vi "SetStreamingFilter.Do.vi"(8 "error in (no error)":errorcluster, 10 "State Variables":T1, 11 "gRPC Request":T12) -> (0 "error out":errorcluster, 2 "State Variables out":T1, 3 "gRPC Response":T13)   [LabVIEW 2025, in "xnet_can_bus_monitor_api_server_do.lvlib"]
uses:
  xnet_can_bus_monitor_api_server_do.lvlib
  xnet_can_bus_monitor_api_server/RPC Messages/ni_xnet_can_bm_api_ErrorInfo.ctl
  xnet_can_bus_monitor_api_server/xnet_can_bus_monitor_api_server.lvlib
  xnet_can_bus_monitor_api_server/RPC Messages/ni_xnet_can_bm_api_SetStreamingFilterReply.ctl
  xnet_can_bus_monitor_api_server/RPC Messages/ni_xnet_can_bm_api_FrameFilter.ctl
  xnet_can_bus_monitor_api_server/RPC Messages/ni_xnet_can_bm_api_DirectionFilter.ctl
  xnet_can_bus_monitor_api_server/RPC Messages/ni_xnet_can_bm_api_FilterInfo.ctl
  xnet_can_bus_monitor_api_server/RPC Messages/ni_xnet_can_bm_api_FdIsoMode.ctl
  xnet_can_bus_monitor_api_server/RPC Messages/ni_xnet_can_bm_api_Termination.ctl
  xnet_can_bus_monitor_api_server/RPC Messages/ni_xnet_can_bm_api_CanMode.ctl
  xnet_can_bus_monitor_api_server/RPC Messages/ni_xnet_can_bm_api_ConnectSettings.ctl
  Types/XNET.InitialSettings.ctl
  Types/StreamProcess.VIRef.ctl
  Types/StreamProcess.Refs.ctl
  Types/MainProcess.StateVariables.ctl
  xnet_can_bus_monitor_api_server/RPC Messages/ni_xnet_can_bm_api_SetStreamingFilterRequest.ctl
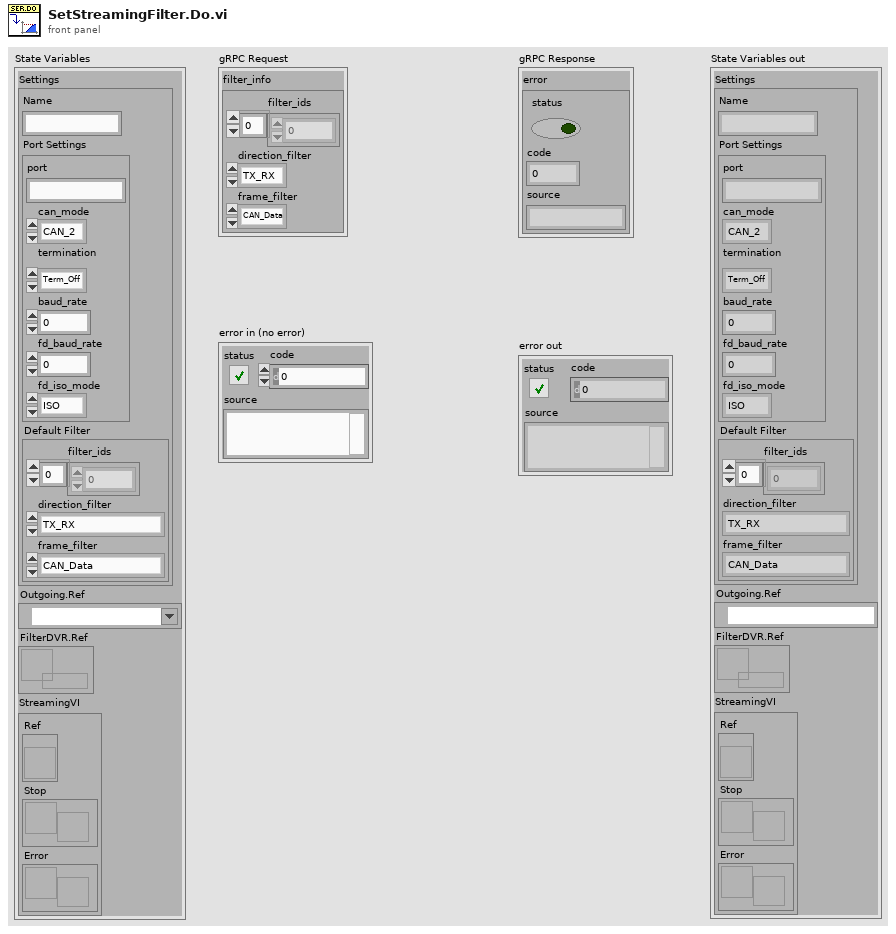
[diagram p1: front panel]
types:
  T1 = typedef "xnet_can_bus_monitor_api_server_do.lvlib/MainProcess.StateVariables.ctl" = cluster{"Settings":T2, "Outgoing.Ref":refnum<k21>, "FilterDVR.Ref":refnum<data-value>, "StreamingVI":T10}
  T2 = typedef "xnet_can_bus_monitor_api_server_do.lvlib/XNET.InitialSettings.ctl" = cluster{"Name":string, "Port Settings":T3, "Default Filter":T7}
  T3 = typedef "xnet_can_bus_monitor_api_server.lvlib/ni_xnet_can_bm_api_ConnectSettings.ctl" = cluster{"port":string, "can_mode":T4, "termination":T5, "baud_rate":u64, "fd_baud_rate":u64, "fd_iso_mode":T6}
  T4 = typedef "xnet_can_bus_monitor_api_server.lvlib/ni_xnet_can_bm_api_CanMode.ctl" = enum32{"CAN_2", "CAN_FD", "CAN_FD_BRS"}
  T5 = typedef "xnet_can_bus_monitor_api_server.lvlib/ni_xnet_can_bm_api_Termination.ctl" = enum32{"Term_Off", "Term_On"}
  T6 = typedef "xnet_can_bus_monitor_api_server.lvlib/ni_xnet_can_bm_api_FdIsoMode.ctl" = enum32{"ISO", "Non_ISO", "ISO_Legacy"}
  T7 = typedef "xnet_can_bus_monitor_api_server.lvlib/ni_xnet_can_bm_api_FilterInfo.ctl" = cluster{"filter_ids":u32[], "direction_filter":T8, "frame_filter":T9}
  T8 = typedef "xnet_can_bus_monitor_api_server.lvlib/ni_xnet_can_bm_api_DirectionFilter.ctl" = enum32{"TX_RX", "RX", "TX"}
  T9 = typedef "xnet_can_bus_monitor_api_server.lvlib/ni_xnet_can_bm_api_FrameFilter.ctl" = enum32{"CAN_Data", "CAN_Remote", "CAN_Bus_Error", "CAN_2_Data", "CAN_FD_Data", "CAN_FD_BRS_Data", "J1939_Data", "Delay", "Log_Trigger", "Start_Trigger", "All"}
  T10 = typedef "xnet_can_bus_monitor_api_server_do.lvlib/StreamProcess.Refs.ctl" = cluster{"Ref":T11, "Stop":refnum<notifier>, "Error":refnum<notifier>}
  T11 = typedef "xnet_can_bus_monitor_api_server_do.lvlib/StreamProcess.VIRef.ctl" = refnum<vi>
  T12 = typedef "xnet_can_bus_monitor_api_server.lvlib/ni_xnet_can_bm_api_SetStreamingFilterRequest.ctl" = cluster{"filter_info":T7}
  T13 = typedef "xnet_can_bus_monitor_api_server.lvlib/ni_xnet_can_bm_api_SetStreamingFilterReply.ctl" = cluster{"error":T14}
  T14 = typedef "xnet_can_bus_monitor_api_server.lvlib/ni_xnet_can_bm_api_ErrorInfo.ctl" = errorcluster
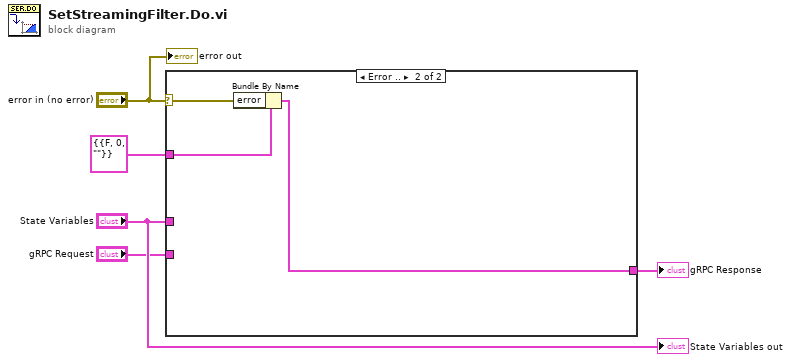
[diagram p0: block diagram]
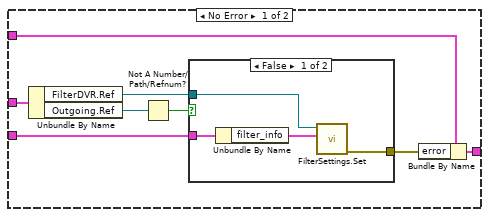
[diagram p2: hidden frame]
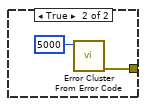
[diagram p3: hidden frame]
diagram:
  n1 = case shown="Error .." "error in (no error)" {
    selector: "error in (no error)" -> [_ w21]
    tunnel: "State Variables" -> [w13 _]
    tunnel: [w10 w20] -> w4
    tunnel: T13 {"error"={"status"=FALSE, "code"=0, "source"=""}} ("Message Data") -> [w9 w22]
    tunnel: "gRPC Request" -> [w7 _]
    frame No Error {
      n2 = Unbundle By Name(w13) -> ("FilterDVR.Ref"=w12:refnum<data-value>, "Outgoing.Ref"=w11:refnum<k21>)
      n3 = Not A Number/Path/Refnum?(number/path/refnum=w11) -> (NaN/Path/Refnum?=w6:bool)
      n4 = case shown="False" w6 {
        tunnel: w7 -> [w16 _]
        tunnel: [w17 w18] -> w8
        tunnel: w12 -> [w14 _]
        frame False {
          n5 = Unbundle By Name(w16) -> ("filter_info"=w15:T7)
          n6 = call "FilterSettings.Set.vi"("Filter"=w15, "FilterDVR.Ref"=w14) -> ("error out"=w17:errorcluster)  [unwired: 9 in]
        }
        frame True {
          n7 = call <vilib>:"Error Cluster From Error Code.vi"("error code (0)"=5000) -> ("error out"=w18:errorcluster)  [unwired: 8 in]
        }
      }
      n8 = Bundle By Name(cluster=w9, "error"=w8) -> (w10:T13)
    }
    frame Error {
      n9 = Bundle By Name(cluster=w22, "error"=w21) -> (w20:T13)
    }
  }
  "gRPC Response" <- w4
  "State Variables out" <- "State Variables"
  "error out" <- "error in (no error)"
